vi "util.convert.u8.to.u64.vi"(11 "unsigned byte array":u8[](array[numeric])) -> (2 "size":i32, 3 "Array":u64[](array[numeric]) format="%.0x")   [LabVIEW 2021]
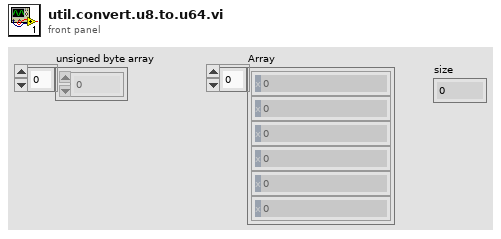
[diagram p1: front panel]
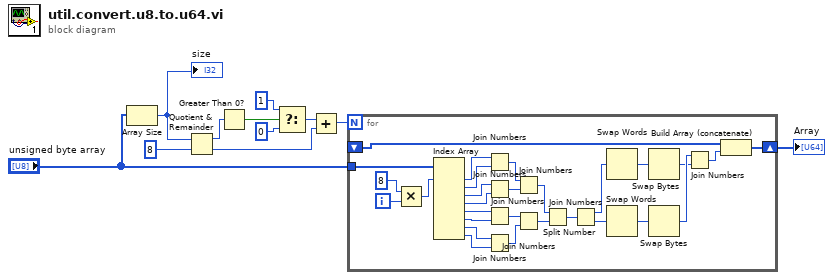
[diagram p0: block diagram]
diagram:
  n1 = Array Size(array="unsigned byte array") -> (size(s)=w4:i32)
  "size" <- w4
  n2 = Quotient & Remainder(x=w4, y=8) -> (x-y*floor(x/y)=w5:i32, floor(x/y)=w10:i32)
  n3 = Greater Than 0?(x=w5) -> (x > 0?=w6:bool)
  n4 = Select(t=1, s=w6, f=0) -> (s? t:f=w8:i32)
  n5 = Add(x=w8, y=w10) -> (x+y=w9:i32)
  n6 = for {
    N: w9 -> [_]
    tunnel: "unsigned byte array" -> [w16]
    shift-right: [w13] -> w2
    shift-left: _ -> [w12]
    i -> [w39]
    n7 = Multiply(x=8, y=w39) -> (x*y=w15:i32)
    n8 = Index Array(array=w16, index #1=w15) -> (element #1=w24:u8, element #2=w25:u8, element #3=w26:u8, element #4=w27:u8, element #5=w28:u8, element #6=w29:u8, element #7=w30:u8, element #8=w31:u8)  [unwired: 7 in]
    n9 = Join Numbers(hi=w24, lo=w25) -> ((hi.lo)=w32:u16)
    n10 = Join Numbers(hi=w26, lo=w27) -> ((hi.lo)=w33:u16)
    n11 = Join Numbers(hi=w28, lo=w29) -> ((hi.lo)=w34:u16)
    n12 = Join Numbers(hi=w30, lo=w31) -> ((hi.lo)=w35:u16)
    n13 = Join Numbers(hi=w32, lo=w33) -> ((hi.lo)=w37:u32)
    n14 = Join Numbers(hi=w34, lo=w35) -> ((hi.lo)=w36:u32)
    n15 = Join Numbers(hi=w37, lo=w36) -> ((hi.lo)=w17:u64)
    n16 = Split Number(x=w17) -> (hi(x)=w23:u32, lo(x)=w22:u32)
    n17 = Swap Words(1:w23) -> (0:w21:u32)
    n18 = Swap Words(1:w22) -> (0:w20:u32)
    n19 = Swap Bytes(anything=w21) -> (byte swapped=w18:u32)
    n20 = Swap Bytes(anything=w20) -> (byte swapped=w19:u32)
    n21 = Join Numbers(hi=w19, lo=w18) -> ((hi.lo)=w14:u64)
    n22 = Build Array (concatenate)(w12, w14) -> (w13:u64[])
  }
  "Array" <- w2
